vi "Verify Combinations.vi"(5 "Label":string, 7 "Options":refnum<class "Options.lvclass">, 8 "error in":errorcluster, 9 "ctl label -> value var[]":map{string, variant[]}(c390), 10 "VI Refnum":refnum<vi>, 11 "TestCase in":refnum<class "TestCase.lvclass">) -> (0 "error out":errorcluster, 3 "TestCase out":refnum<class "TestCase.lvclass">)   [LabVIEW 2026, in "VITester.Extension.lvlib"]
doc: "This is similar to the verify parameterized (in fact it calls it behind the scenes). Instead of specifying each set of parameters, you specify a single map which maps each control label to an array of variant values (there is a utility vi, \"array to array of variants.vim) to assist with this. From this, the verify function calculates each set of parameters from all the possible combinations and verifyies each combination."
uses:
  VITester.Extension.lvlib
  <vilib>/Addons/_JKI Toolkits/VI Tester/TestCase.llb/TestCase.lvclass
  Approval Tests/Options/Options.lvclass
  Approval Tests/Options/Options.lvclass/Options.ctl
  Approval Tests/Naming Data/Naming Data.lvclass/Naming Data.ctl
  Approval Tests/Naming Data/Read Test VI Name.vi
  Approval Tests/Naming Data/Write Test VI Name.vi
  Approval Tests/Approval Tests.lvlib
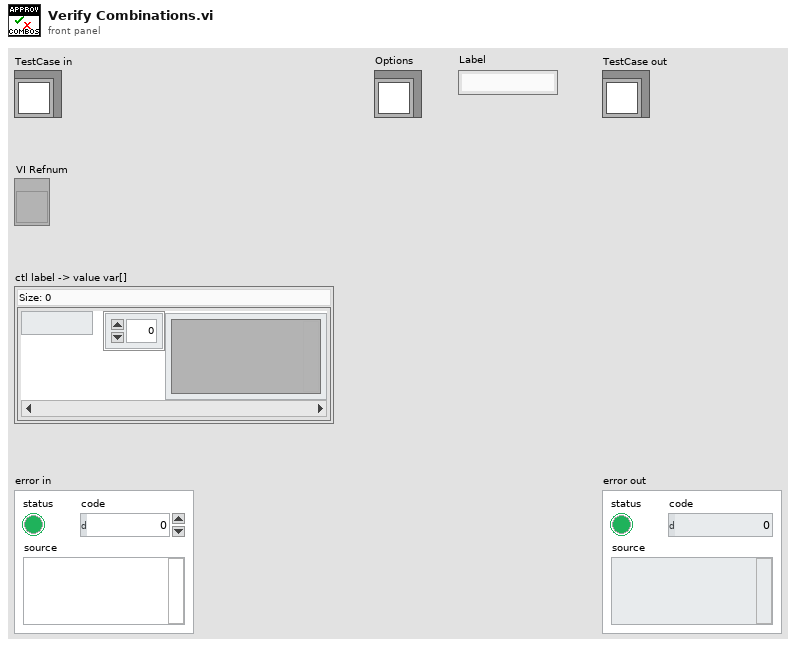
[diagram p1: front panel]
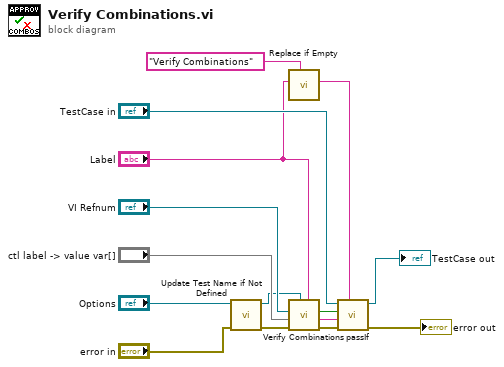
[diagram p0: block diagram]
diagram:
  n1 = call "Update Test Name if Not Defined.vi"("error in"="error in", "Options in"="Options") -> ("error out"=w12:errorcluster, "Options out"=w4:refnum<class "Options.lvclass">)  [unwired: 8 in]
  n2 = call "Replace if Empty.vi"("if empty"="Verify Combinations", "Text in"="Label") -> ("Text out"=w1:string)  [unwired: 9 in]
  n3 = call "Verify Combinations.vi"("Label"="Label", "Approval Tests.lvlib:Options.lvclass"=w4, "error in"=w12, "ctl label -> value var[]"="ctl label -> value var[]", "VI Refnum"="VI Refnum") -> ("error out"=w14:errorcluster, "Failure Message"=w8:string, "Passed?"=w9:bool)  [unwired: 4 in]
  n4 = call-dynamic "passIf.vi"("custom report message (\"\")"=w1, "error in (no error)"=w14, "message (\"\")"=w8, "pass"=w9, "TestCase in"="TestCase in") -> ("error out"=→"error out":errorcluster, "TestCase out"=→"TestCase out":refnum<class "TestCase.lvclass">)  [unwired: 5 in]
